vi "File.Check File Type, Option to Read from Zip.vi"(7 "TempFolder":path=path "c:/MTE/Data/Temp/Unzip", 8 "error in (no error)":errorcluster, 11 "Data File":path) -> (0 "error out":errorcluster, 1 "Unzipped":bool, 2 "Valid":bool, 3 "Unzipped File":path)   [LabVIEW 2024]
uses:
  <vilib>/zip/NI_Unzip.lvlib
  File Utils.lvlib
panel:
  in  "File Extension":string="json"
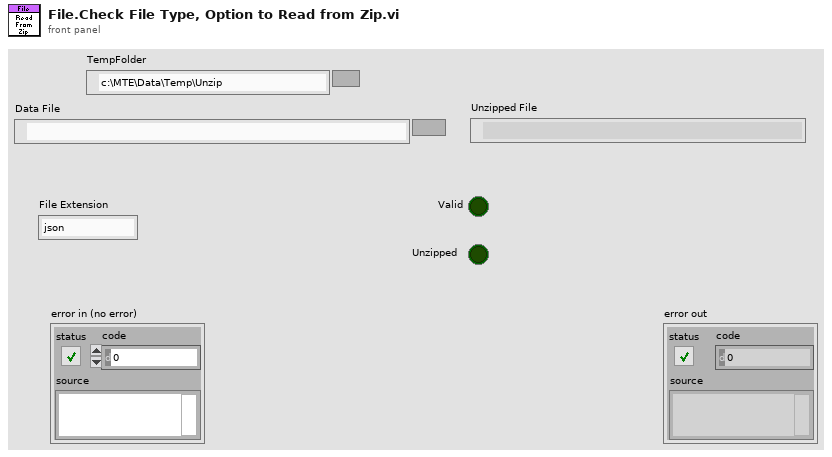
[diagram p1: front panel]
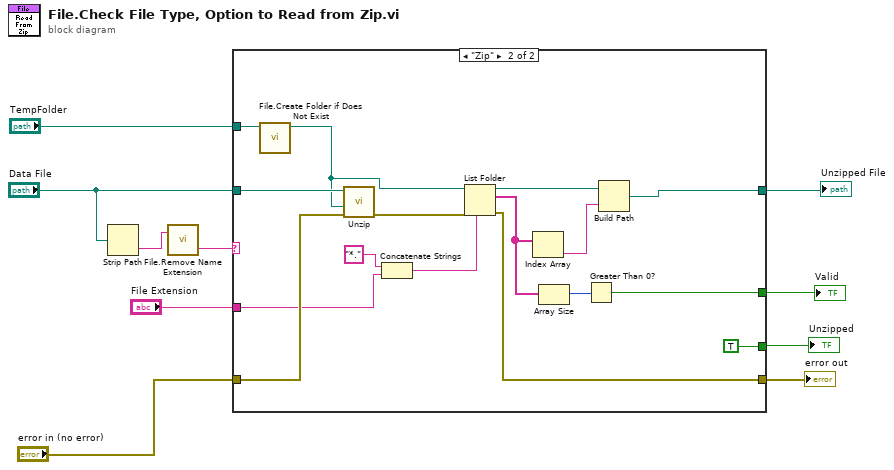
[diagram p0: block diagram]
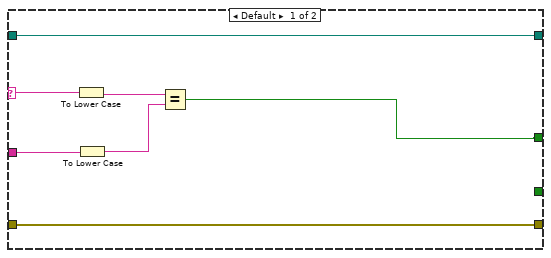
[diagram p2: hidden frame]
diagram:
  n1 = Strip Path(path="Data File") -> (name=w10:string)  [unwired: 1 out]
  n2 = call "File.Remove Name Extension.vi"("File Name"=w10) -> ("Ext"=w9:string)  [unwired: 1 in, 1 out]
  n3 = case shown="\"Zip\"" w9 {
    selector: w9 -> [w15 _]
    tunnel: [w17 w29] -> w4
    tunnel: "Data File" -> [w17 w33]
    tunnel: "TempFolder" -> [_ w19]
    tunnel: [w11 w26] -> w6
    tunnel: [_ TRUE] -> w5
    tunnel: "error in (no error)" -> [w16 w24]
    tunnel: [w16 w23] -> w2
    tunnel: "File Extension" -> [w14 w21]
    frame Default {
      n4 = To Lower Case(string=w15) -> (all lower case string=w12:string)
      n5 = To Lower Case(string=w14) -> (all lower case string=w13:string)
      n6 = Equal?(x=w12, y=w13) -> (x = y?=w11:bool)
    }
    frame "Zip" {
      n7 = call "File.Create Folder if Does Not Exist.vi"("Path"=w19) -> ("Dup Path"=w18:path)  [unwired: 8 in, 2 out]
      n8 = call <vilib>:"Unzip.vi"("error in (no error)"=w24, "Target directory (same as Zip file if empty)"=w18, "Zip file"=w33) -> ("error out"=w32:errorcluster)  [unwired: 6 in, 2 out]
      n9 = Concatenate Strings("*." ("pattern"), w21) -> (w20:string)
      n10 = List Folder(path=w18, pattern=w20, error in=w32) -> (path out=w30:path, filenames=w28:string[], error out=w23:errorcluster)  [unwired: 1 in, 1 out]
      n11 = Index Array(array=w28) -> (element=w31:string)  [unwired: 1 in]
      n12 = Array Size(array=w28) -> (size(s)=w27:i32)
      n13 = Greater Than 0?(x=w27) -> (x > 0?=w26:bool)
      n14 = Build Path(base path=w30, name or relative path=w31) -> (appended path=w29:path)
    }
  }
  "Valid" <- w6
  "Unzipped" <- w5
  "Unzipped File" <- w4
  "error out" <- w2
